vi "DesiredRow2DesiredParameters.vi"(0 "DesiredStatRow":string[](array[string])) -> (4 "DesiredParameters":T1, 8 "Controller?":bool)   [LabVIEW 2013]
uses:
  TypeDef/Command Cluster.ctl
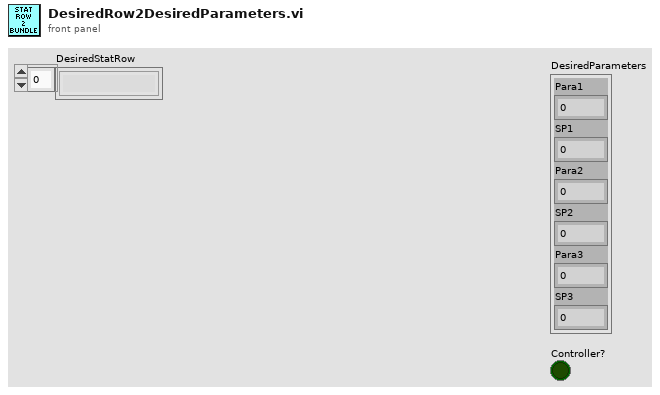
[diagram p1: front panel]
types:
  T1 = typedef "Command Cluster.ctl" = cluster{"Para1":i32, "SP1":dbl, "Para2":i32, "SP2":dbl, "Para3":i32, "SP3":dbl}
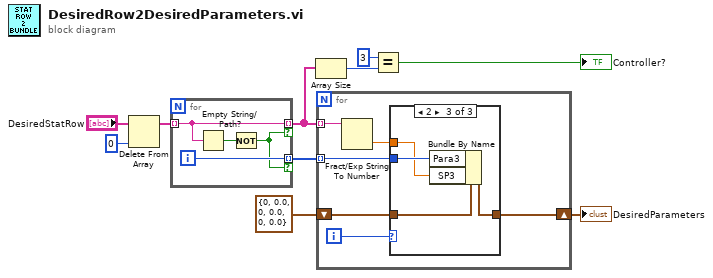
[diagram p0: block diagram]
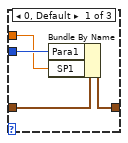
[diagram p2: hidden frame]
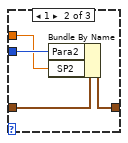
[diagram p3: hidden frame]
diagram:
  n1 = Delete From Array(array="DesiredStatRow", index=0) -> (array with subset deleted=w8:string[])  [unwired: 1 in, 1 out]
  n2 = for {
    tunnel: w8 -> [w14] mode=indexing
    tunnel: [w14] -> w7 mode=indexing if=w11
    tunnel: [w12] -> w6 mode=indexing if=w11
    i -> [w12]
    n3 = Empty String/Path?(string/path=w14) -> (empty?=w13:bool)
    n4 = Not(x=w13) -> (.not. x?=w11:bool)
  }
  n5 = Array Size(array=w7) -> (size(s)=w5:i32)
  n6 = for {
    tunnel: w7 -> [w16] mode=indexing
    tunnel: w6 -> [w17] mode=indexing
    shift-right: [w18] -> w1
    shift-left: T1 {"Para1"=0, "SP1"=0.0, "Para2"=0, "SP2"=0.0, "Para3"=0, "SP3"=0.0} ("DesiredParameters") -> [w19]
    i -> [w20]
    n7 = Fract/Exp String To Number(string=w16) -> (number=w15:dbl)  [unwired: 3 in, 1 out]
    n8 = case shown="2" w20 {
      tunnel: w19 -> [w24 w28 w32]
      tunnel: [w23 w27 w31] -> w18
      tunnel: w17 -> [w22 w26 w30]
      tunnel: w15 -> [w21 w25 w29]
      frame 0, Default {
        n9 = Bundle By Name(cluster=w24, "Para1"=w22, "SP1"=w21) -> (w23:T1)
      }
      frame 1 {
        n10 = Bundle By Name(cluster=w28, "Para2"=w26, "SP2"=w25) -> (w27:T1)
      }
      frame 2 {
        n11 = Bundle By Name(cluster=w32, "Para3"=w30, "SP3"=w29) -> (w31:T1)
      }
    }
  }
  "DesiredParameters" <- w1
  n12 = Equal?(x=3, y=w5) -> (x = y?=→"Controller?":bool)
